vi "normalize_vector.vi"(1 "Input vector":dbl[](array[numeric])) -> (0 "Normalized vector":dbl[](array[numeric]))   [LabVIEW 2015]
doc: "Normalizes 1D vector of any size"
panel:
  out "norm":dbl
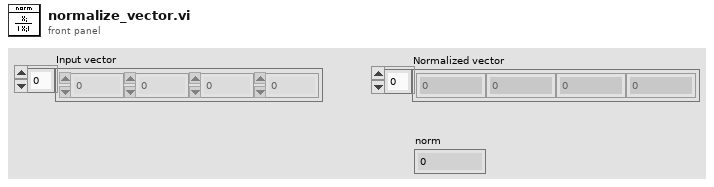
[diagram p1: front panel]
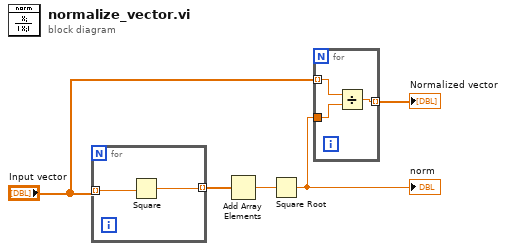
[diagram p0: block diagram]
diagram:
  n1 = for {
    tunnel: "Input vector" -> [w7] mode=indexing
    tunnel: [w6] -> w5 mode=indexing
    n2 = Square(x=w7) -> (x^2=w6:dbl)
  }
  n3 = Add Array Elements(numeric array=w5) -> (sum=w4:dbl)
  n4 = Square Root(x=w4) -> (sqrt(x)=w2:dbl)
  "norm" <- w2
  n5 = for {
    tunnel: "Input vector" -> [w10] mode=indexing
    tunnel: w2 -> [w9]
    tunnel: [w8] -> w1 mode=indexing
    n6 = Divide(x=w10, y=w9) -> (x/y=w8:dbl)
  }
  "Normalized vector" <- w1
